vi "config_parser.vi"(4 "error in":errorcluster, 5 "key":string="connection_table_h5", 6 "section":string="paths", 7 "path":path=path "C:/labconfig/bec-spinor-imaging.ini") -> (0 "error out":errorcluster, 3 "result":string)   [LabVIEW 2010]
uses:
  <vilib>/regexp/Match Regular Expression.xnode
  <vilib>/Utility/config.llb/Read Key (String).vi
  <vilib>/Utility/config.llb/NI_LVConfig.lvlib
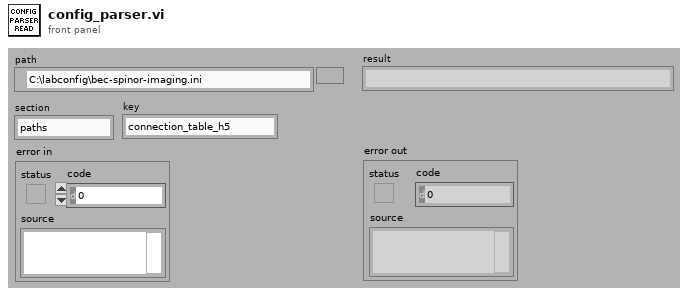
[diagram p1: front panel]
types:
  T1 = typedef "NI_LVConfig.lvlib/Config Data RefNum.ctl" = refnum<k1>
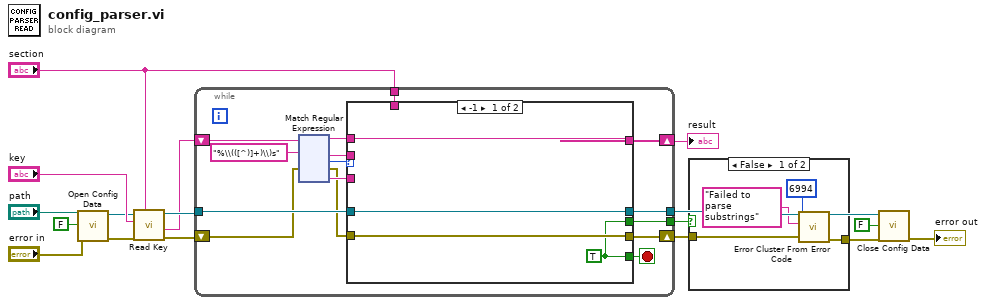
[diagram p0: block diagram]
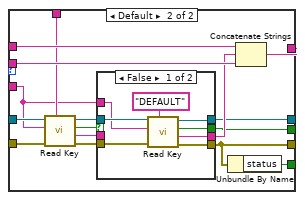
[diagram p3: hidden frame]
diagram:
  n1 = call <vilib>:"Open Config Data.vi"("error in (no error)"="error in", "create file if necessary (T)"=FALSE, "configuration file path"="path") -> ("error out"=w8:errorcluster, "refnum"=w9:T1)  [unwired: 6 in, 1 out]
  n2 = call-poly <vilib>:"Read Key.vi"("section"="section", "error in (no error)"=w8, "key"="key", "refnum"=w9) -> ("error out"=w7:errorcluster, "value"=w11:string, "refnum out"=w15:T1)  [unwired: 4 in, 1 out]
  n3 = while {
    tunnel: w15 -> [w27]
    tunnel: [w26] -> w14
    tunnel: "section" -> [w25]
    shift-right: [w24] -> w12
    shift-left: w11 -> [w32]
    shift-right: [w19] -> w4
    shift-left: w7 -> [w21]
    tunnel: [w18] -> w5
    stop <- w22 stop-if-true
    n4 = xnode "Match Regular Expression"("input string"=w32, "regular expression"="%\\(([^)]+)\\)s", "error in"=w21) -> ("before match"=w30:string, "after match"=w29:string, "offset past match"=w23:i32, "error out"=w20:errorcluster, "submatch 1"=w28:string)  [unwired: 3 in, 1 out]
    n5 = case shown="-1" w23 {
      tunnel: w30 -> [w35 w52]
      tunnel: w29 -> [_ w51]
      tunnel: w28 -> [_ w43]
      tunnel: w27 -> [w36 w50]
      tunnel: [w36 w42] -> w26
      tunnel: w25 -> [_ w49]
      tunnel: [w35 w48] -> w24
      tunnel: [w33 w37] -> w22
      tunnel: w20 -> [w34 w41]
      tunnel: [w34 w38] -> w19
      tunnel: [w33 w39] -> w18
      frame -1 {
        w33 = TRUE
      }
      frame Default {
        n6 = call-poly <vilib>:"Read Key.vi"("section"=w49, "error in (no error)"=w41, "key"=w43, "refnum"=w50) -> ("error out"=w40:errorcluster, "value"=w46:string, "found?"=w47:bool, "refnum out"=w45:T1)  [unwired: 4 in]
        n7 = case shown="False" w47 {
          selector: w47 -> [_ w61]
          tunnel: w46 -> [_ w64]
          tunnel: w45 -> [w60 w63]
          tunnel: [w59 w64] -> w44
          tunnel: w43 -> [w58 _]
          tunnel: [w56 w63] -> w42
          tunnel: w40 -> [w55 w62]
          tunnel: [w54 w62] -> w38
          tunnel: [w53 w61] -> w39
          frame False {
            n8 = call-poly <vilib>:"Read Key.vi"("section"="DEFAULT", "error in (no error)"=w55, "key"=w58, "refnum"=w60) -> ("error out"=w54:errorcluster, "value"=w59:string, "found?"=w53:bool, "refnum out"=w56:T1)  [unwired: 4 in]
          }
          frame True {
          }
        }
        n9 = Unbundle By Name(w38) -> ("status"=w37:bool)
        n10 = Concatenate Strings(w52, w44, w51) -> (w48:string)
      }
    }
  }
  "result" <- w12
  n11 = case shown="False" w5 {
    tunnel: w4 -> [w181 w182]
    tunnel: [w180 w182] -> w3
    frame False {
      n12 = call <vilib>:"Error Cluster From Error Code.vi"("error in (no error)"=w181, "error message (\"\")"="Failed to parse substrings" ("error message (\"\")"), "error code (0)"=6994) -> ("error out"=w180:errorcluster)  [unwired: 6 in]
    }
    frame True {
    }
  }
  n13 = call <vilib>:"Close Config Data.vi"("error in (no error)"=w3, "write file if changed (T)"=FALSE, "refnum"=w14) -> ("error out"=→"error out":errorcluster)  [unwired: 7 in, 1 out]
